vi "testext.vi"() -> ()   [LabVIEW 2011]
uses:
  <vilib>/vision/NI_Vision_Development_Module.lvlib
panel:
  in  "Array":i32[](array[numeric])
  in  "Global Rectangle 2":i32[](array[numeric])
  out "Global Rectangle":i32[](array[numeric])
  out "New Image":T1(plugin-control)
  out "Image Dst Out":T1(plugin-control)
  in  "stop":bool
  in  "Image Pixels (Float)":sgl[][](array[numeric]) format="%.2f"
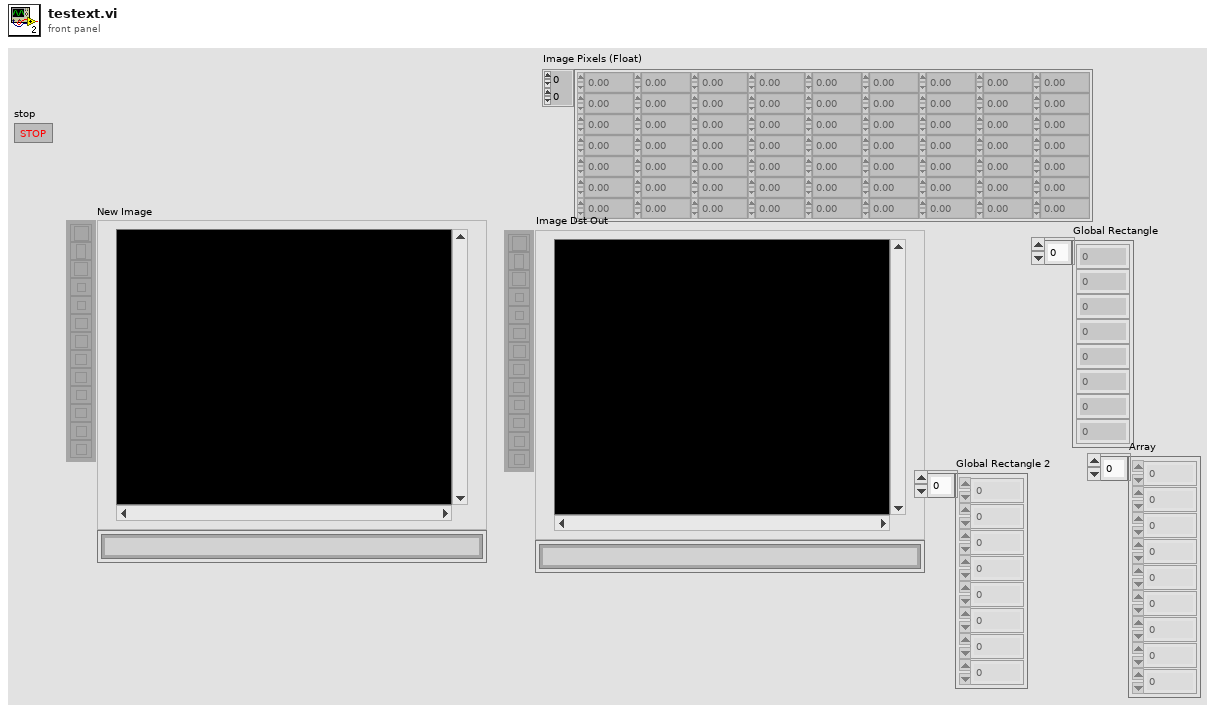
[diagram p1: front panel]
types:
  T1 = typedef "IMAQ Image.ctl" = refnum<image>
  T2 = typedef "Image Type" = u32
  T3 = cluster{"Global Rectangle":i32[], "Contours":cluster{"Contour Type":u32, "ROI Type":u32, "Points":i32[]}[]}
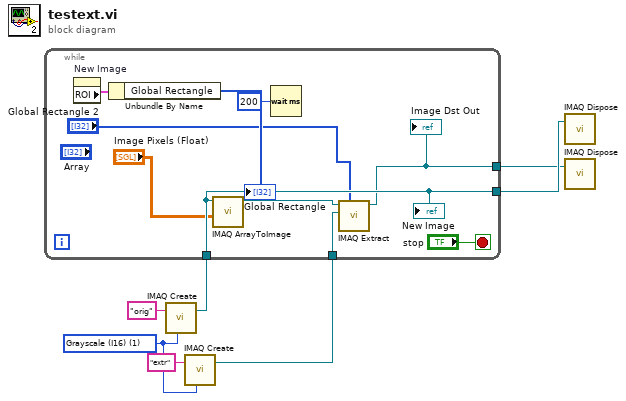
[diagram p0: block diagram]
diagram:
  w4 = T2 1 items=["Grayscale (U8)", "Grayscale (I16)", "Grayscale (SGL)", "Complex (CSG)", "RGB (U32)", "HSL (U32)", "RGB (U64)", "Grayscale (U16)"] ("Image Type")
  n1 = call "IMAQ Create"("Image Name"="orig", "Image Type"=w4) -> ("New Image"=w6:T1)  [unwired: 3 in, 1 out]
  n2 = call "IMAQ Create"("Image Name"="extr", "Image Type"=w4) -> ("New Image"=w5:T1)  [unwired: 3 in, 1 out]
  n3 = while {
    tunnel: w6 -> [w14]
    tunnel: w5 -> [w16]
    tunnel: [w14] -> w2
    tunnel: [w12] -> w1
    stop <- "stop" stop-if-true
    n4 = property on="New Image" class="ImageControl"() -> ("ROI"=w10:T3)  [unwired: 2 in, 2 out]
    n5 = Unbundle By Name(w10) -> ("Global Rectangle"=→"Global Rectangle":i32[])
    n6 = call "IMAQ ArrayToImage"("Image Pixels (I16)"="Image Pixels (Float)", "Image"=w14) -> ("Image Out"=w17:T1)  [unwired: 8 in, 1 out]
    n7 = Wait (ms)(milliseconds to wait=u32 200) -> ()  [unwired: 1 out]
    n8 = call "IMAQ Extract"("Optional Rectangle"="Global Rectangle 2", "Image Dst"=w16, "Image Src"=w17) -> ("Image Dst Out"=w12:T1)  [unwired: 7 in, 1 out]
    "Image Dst Out" <- w12
    "New Image" <- w14
  }
  n9 = call "IMAQ Dispose"("Image"=w2) -> ()  [unwired: 5 in, 1 out]
  n10 = call "IMAQ Dispose"("Image"=w1) -> ()  [unwired: 5 in, 1 out]
